vi "Z-Scan.vi"() -> ()   [LabVIEW 2010]
uses:
  <vilib>/Utility/error.llb/DialogType.ctl
  <vilib>/express/express arith-compare/Formula/XNode/ExpressFormulaBlockNode.xnode
  <vilib>/DAQmx/read.llb/DAQmx Read (Analog 1D Wfm NChan NSamp).vi
  <vilib>/DAQmx/create/channels.llb/DAQmx Create Channel (AI-Voltage-Basic).vi
  <vilib>/DAQmx/configure/timing.llb/DAQmx Timing (Sample Clock).vi
  <vilib>/DAQmx/configure/trigger.llb/DAQmx Start Trigger (Digital Edge).vi
  <vilib>/daqmx/miscellaneous.llb/DAQmx Fill In Error Info.vi
  <vilib>/express/express shared/transition.llb/Dynamic To Waveform Array.vi
  <vilib>/express/express shared/transition.llb/Waveform Array To Dynamic.vi
  <vilib>/express/express arith-compare/Formula/Block/exnFormulaBlock how many pts in the wave.vi
  <vilib>/express/express shared/ex_Modify Signal Name.vi
  Program Files (x86)/National Instruments/LabVIEW 2010/resource/objmgr/daqmx.rc
panel:
  in  "lower threshold":dbl
  in  "upper threshold":dbl
  out "Ioa":cluster{dbl[], dbl[]}(graph)
  in  "stop 11":bool
  out "Ica":cluster{dbl[], dbl[]}(graph)
  out "Ioca":cluster{dbl[], dbl[]}(graph)
  in  "x max (mm)":dbl=500.0
  in  "x step (mm)":dbl=5.0
  in  "N":i32=1000
  in  "x min (mm)":dbl=-0.5
  in  "error in":errorcluster
  out "Signal 2":waveform(dbl)[](graph)
  in  "Ring":u16(ring)=1 items=["Ref", "OA", "CA"]
  in  "stop 2":bool
  out "Trigger delay":dbl format="%#_6e"
  in  "Signal":tag="Dev2/ai0"
  in  "Minimum value (V)":dbl=-5.0
  in  "Maximum value (V)":dbl=10.0
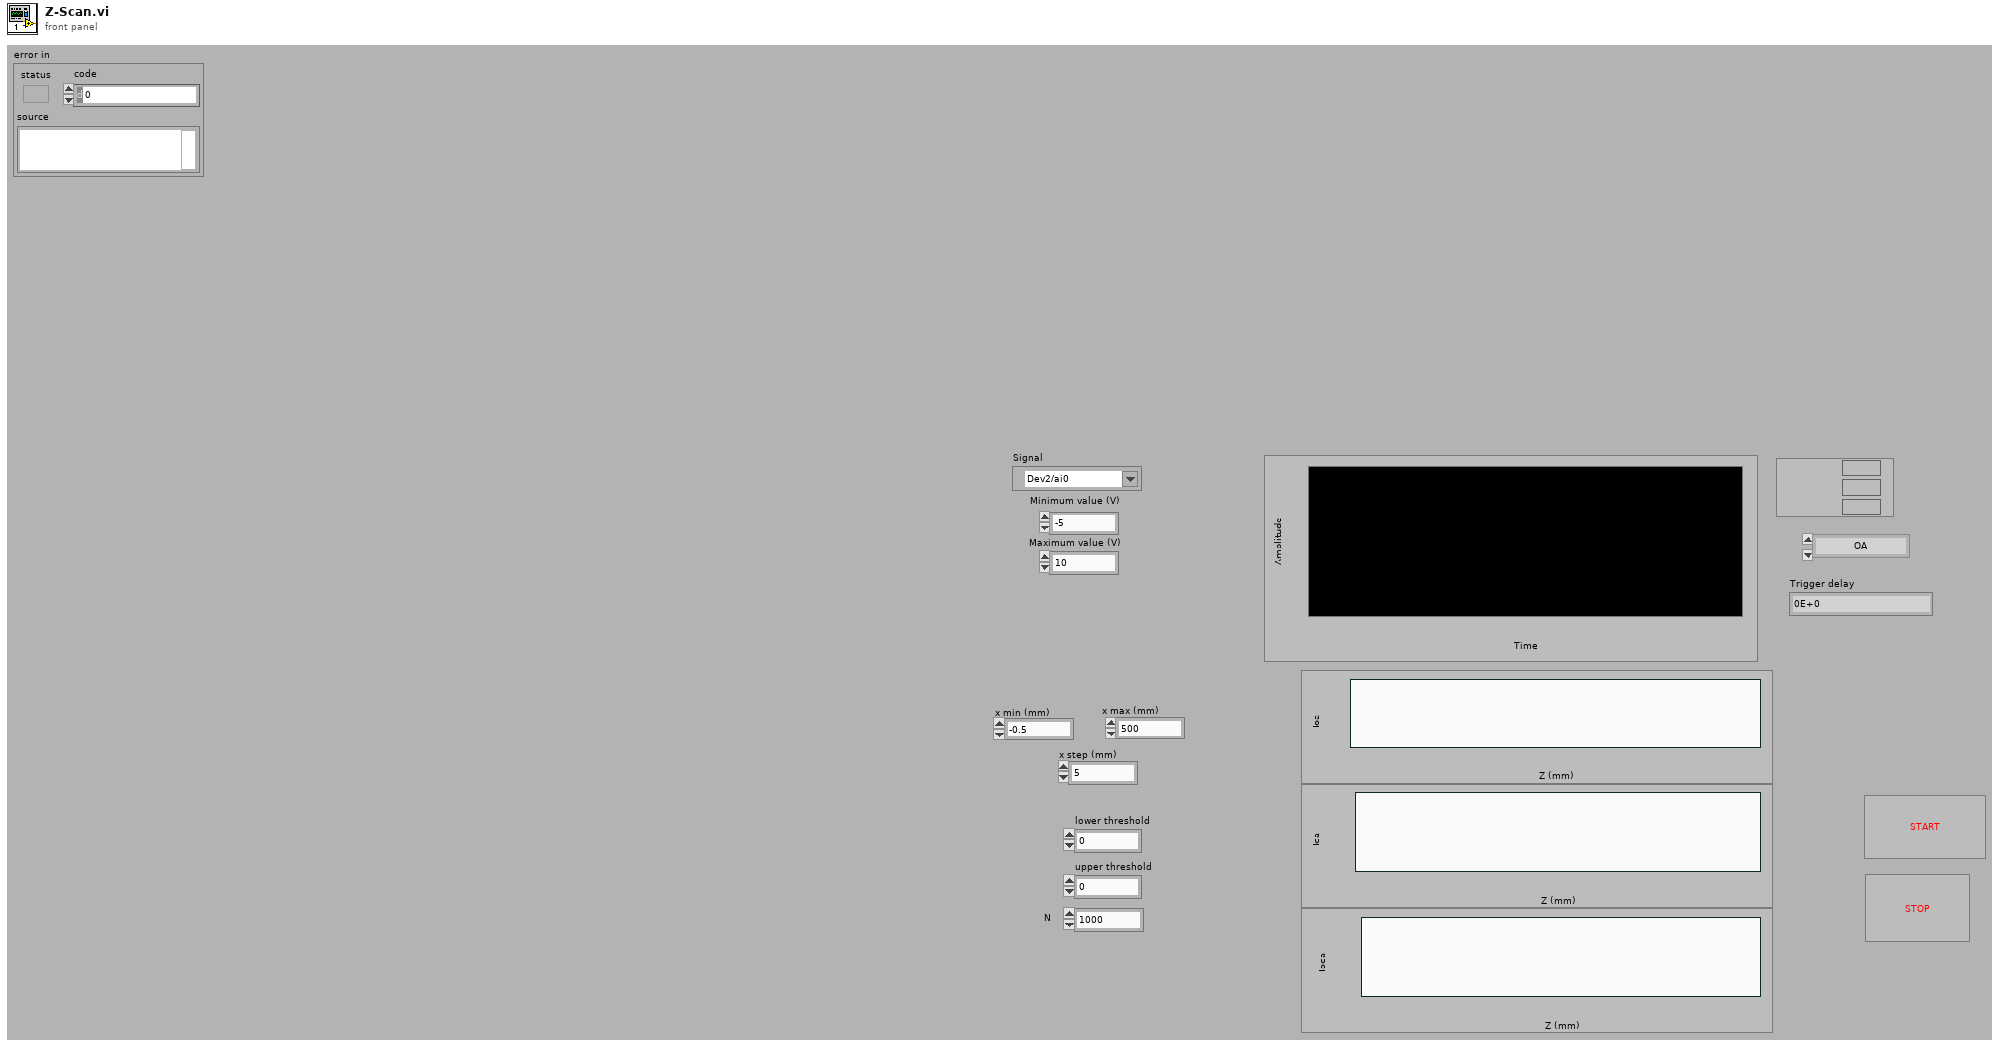
[diagram p1: front panel]
types:
  T1 = enum16{"open", "replace", "create", "open or create", "replace or create", "replace or create with confirmation"}
  T2 = typedef "DialogType.ctl" = u16
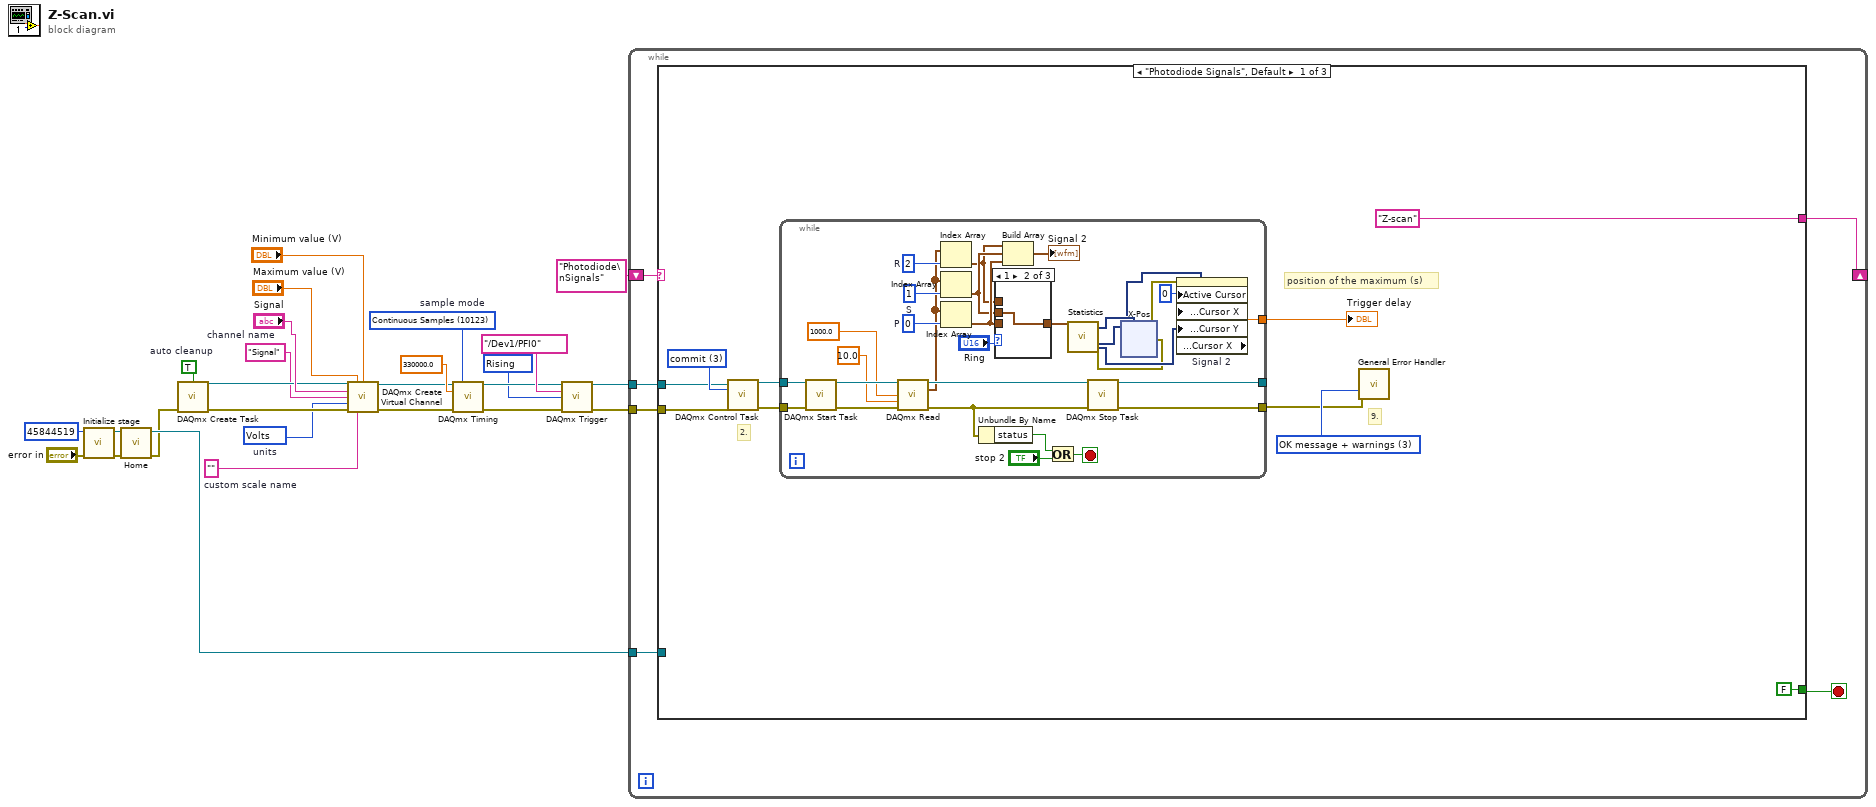
[diagram p0: block diagram]
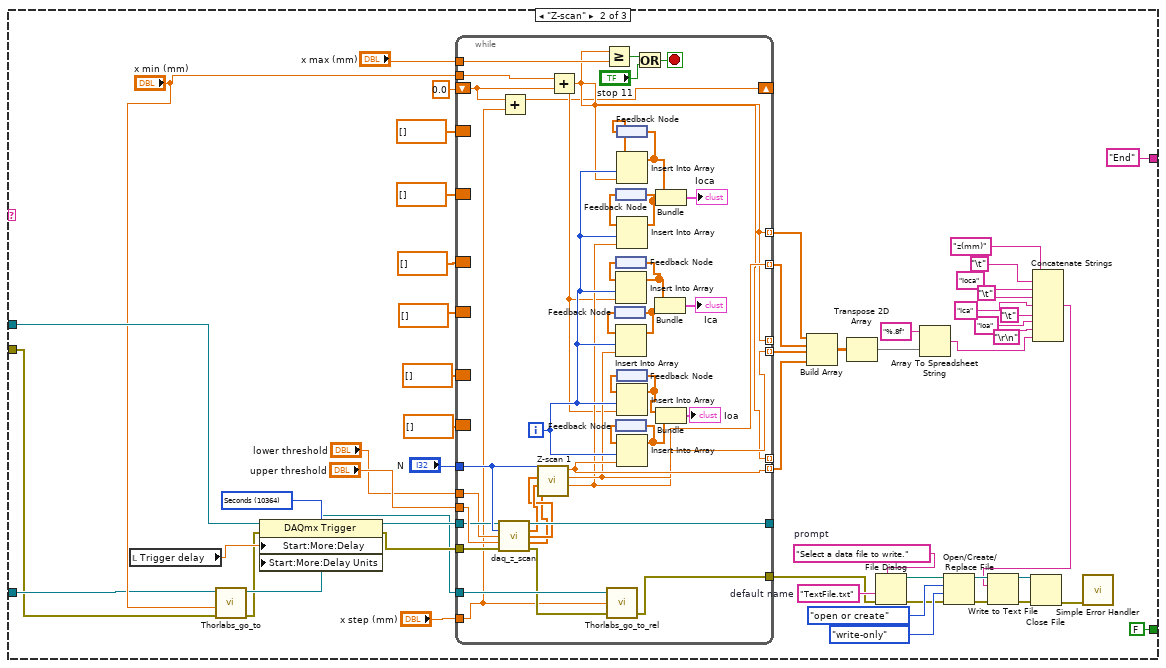
[diagram p4: hidden frame]
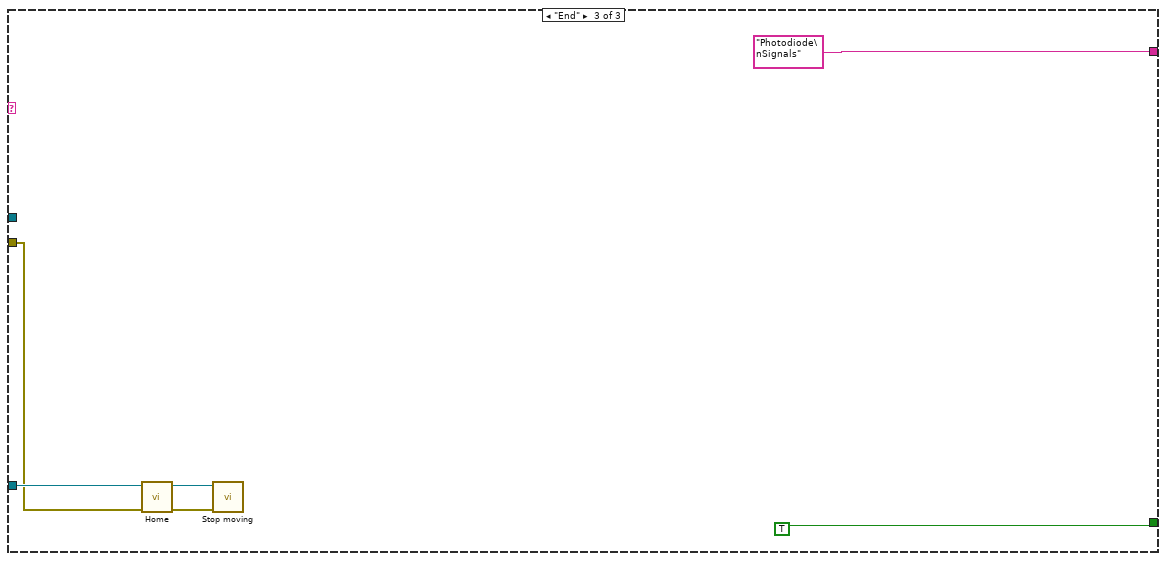
[diagram p5: hidden frame]
diagram:
  w15 = 10280 items=["Rising"=10280, "Falling"=10171] ("Trigger edge")
  w17 = 10123 items=["Finite Samples"=10178, "Continuous Samples"=10123, "Hardware Timed Single Point"=12522]  # sample mode
  w9 = 10348 items=["Volts"=10348, "From Custom Scale"=10065]  # units
  w10 = "Signal"  # channel name
  w8 = ""  # custom scale name
  w11 = TRUE  # auto cleanup
  n1 = call <instrlib>:"Initialize stage.vi"("error in (no error)"="error in", "HWSerialNum"=45844519) -> ("error out"=w6:errorcluster, "reference out"=w5:refnum<k7>)  [unwired: 8 in]
  n2 = call <instrlib>:"Home.vi"("error in"=w6, "in"=w5) -> ("error out"=w1:errorcluster, "out"=w2:refnum<k7>)  [unwired: 8 in]
  n3 = call <vilib>:"DAQmx Create Task.vi"("auto cleanup"=w11, "error in"=w1) -> ("task out"=w12:refnum<k21>, "error out"=w14:errorcluster)  [unwired: 12 in]
  n4 = call-poly <vilib>:"DAQmx Create Virtual Channel.vi"("task in"=w12, "maximum value"="Maximum value (V)", "minimum value"="Minimum value (V)", "physical channels"="Signal", "name to assign"=w10, "units"=w9, "error in"=w14, "custom scale name"=w8) -> ("task out"=w22:refnum<k21>, "error out"=w23:errorcluster)  [unwired: 6 in]
  n5 = call-poly <vilib>:"DAQmx Timing.vi"("task/channels in"=w22, "sample mode"=w17, "rate"=330000.0, "error in"=w23) -> ("task out"=w16:refnum<k21>, "error out"=w19:errorcluster)  [unwired: 10 in]
  n6 = call-poly <vilib>:"DAQmx Trigger.vi"("task/channels in"=w16, "source"=tag "/Dev1/PFI0", "edge"=w15, "error in"=w19) -> ("task out"=w26:refnum<k21>, "error out"=w25:errorcluster)  [unwired: 10 in]
  n7 = while {
    shift-right: [w31] -> _
    shift-left: "Photodiode\nSignals" -> [w32]
    tunnel: w26 -> [w30]
    tunnel: w25 -> [w29]
    tunnel: w2 -> [w27]
    stop <- w28 stop-if-true
    n8 = case shown="\"Photodiode Signals\", Default" w32 {
      tunnel: ["Z-scan" "End" "Photodiode\nSignals"] -> w31
      tunnel: w30 -> [w35 w252 _]
      tunnel: w29 -> [w34 w227 w310]
      tunnel: [FALSE FALSE TRUE] -> w28
      tunnel: w27 -> [_ w229 w312]
      frame "Photodiode Signals", Default {
        w41 = T2 3 items=["no dialog", "OK message", "continue or stop message", "OK message + warnings", "continue/stop + warnings"] ("type of dialog (OK msg:1)")
        w36 = 3 items=["verify"=2, "reserve"=4, "commit"=3, "unreserve"=5, "abort"=6] ("action")
        # "position of the maximum (s)"
        # "9."
        # "2."
        n9 = call <vilib>:"DAQmx Control Task.vi"("task/channels in"=w35, "action"=w36, "error in"=w34) -> ("task out"=w37:refnum<k21>, "error out"=w38:errorcluster)  [unwired: 11 in]
        n10 = while {
          tunnel: w37 -> [w73]
          tunnel: w38 -> [w72]
          tunnel: [w71] -> w40
          tunnel: [w49] -> _
          tunnel: [w48] -> w39
          stop <- w44 stop-if-true
          w64 = 0  # P
          w65 = 1  # S
          w66 = 2  # R
          n11 = call <vilib>:"DAQmx Start Task.vi"("task/channels in"=w73, "error in"=w72) -> ("task out"=w70:refnum<k21>, "error out"=w69:errorcluster)  [unwired: 12 in]
          n12 = call-poly <vilib>:"DAQmx Read.vi"("task/channels in"=w70, "number of samples per channel"=1000.0 ("Samples/channel"), "timeout"=10.0, "error in"=w69) -> ("task out"=w68:refnum<k21>, "data"=w63:waveform(dbl)[], "error out"=w46:errorcluster)  [unwired: 9 in]
          n13 = Index Array(array=w63, index=w66) -> (element=w55:waveform(dbl))
          n14 = Index Array(array=w63, index=w65) -> (element=w56:waveform(dbl))
          n15 = Index Array(array=w63, index=w64) -> (element=w58:waveform(dbl))
          n16 = Unbundle By Name(w46) -> ("status"=w47:bool)
          n17 = case shown="1" "Ring" {
            tunnel: w58 -> [w213 _ _]
            tunnel: [w213 w214 w215] -> w57
            tunnel: w56 -> [_ w214 _]
            tunnel: w55 -> [_ _ w215]
            frame 0, Default {
            }
            frame 1 {
            }
            frame 2 {
            }
          }
          n18 = Build Array(w55, w56, w58) -> (→"Signal 2":waveform(dbl)[])
          n19 = Or(x=w47, y="stop 2") -> (x .or. y?=w44:bool)
          n20 = call "Statistics"("Signals"=w57) -> ("First Time"=w60:dynamicdata, "Time of Maximum"=w61:dynamicdata, "Maximum"=w59:dynamicdata, "error out"=w54:errorcluster)  [unwired: 21 in, 2 out]
          n21 = call <vilib>:"DAQmx Stop Task.vi"("task/channels in"=w68, "error in"=w46) -> ("task out"=w49:refnum<k21>, "error out"=w48:errorcluster)  [unwired: 12 in]
          n22 = xnode "X-Pos"("TimeMax"=w61, "1stTime"=w60, "error in (no error)"=w54) -> ("Result"=w50:dynamicdata, "error out"=w53:errorcluster)
          n23 = property on="Signal 2" class="WFGraph (strict)"(error in=w53, "Active Cursor"=u32 0, "Cursor.Cursor Position:Cursor X"=w50, "Cursor.Cursor Position:Cursor Y"=w59) -> ("Cursor.Cursor Position:Cursor X"=w71:dbl)  [unwired: 1 in, 2 out]
        }
        "Trigger delay" <- w40
        n24 = call <vilib>:"General Error Handler.vi"("type of dialog (OK msg:1)"=w41, "error in (no error)"=w39) -> ()  [unwired: 9 in, 5 out]
      }
      frame "Z-scan" {
        w243 = "TextFile.txt"  # default name
        w244 = "Select a data file to write."  # prompt
        w255 = 10364 items=["Sample Clock Periods"=10286, "Seconds"=10364, "Ticks"=10304] ("Start.DelayUnits")
        n25 = local read "Trigger delay"() -> (w251:dbl)
        n26 = call <userlib>:"Thorlabs_go_to.vi"("error in (no error)"=w227, "Target position (mm)"="x min (mm)", "MG17Motor in"=w229) -> ("error out"=w226:errorcluster, "MG17Motor out"=w228:refnum<k7>)  [unwired: 6 in, 1 out]
        n27 = property class="DAQmx Trigger"(reference=w252, error in=w226, "Start:More:Delay"=w251, "Start:More:Delay Units"=w255) -> (reference out=w254:refnum<k21>, error out=w253:errorcluster)
        n28 = while {
          tunnel: "x max (mm)" -> [w303]
          tunnel: [w275] -> _ mode=indexing
          tunnel: [w296] -> w234 mode=indexing
          tunnel: [w271] -> w238
          tunnel: [w298] -> _
          tunnel: "x min (mm)" -> [w299]
          tunnel: "x step (mm)" -> [w269]
          tunnel: w228 -> [w295]
          tunnel: "N" -> [w297]
          shift-right: [w270] -> _
          shift-left: 0.0 -> [w292]
          border: dbl[] [] -> [_]
          border: dbl[] [] -> [_]
          tunnel: w253 -> [w273]
          tunnel: "upper threshold" -> [w294]
          tunnel: w254 -> [w293]
          border: dbl[] [] -> [_]
          border: dbl[] [] -> [_]
          border: dbl[] [] -> [_]
          border: dbl[] [] -> [_]
          tunnel: [w277] -> w235 mode=indexing
          tunnel: [w275] -> _ mode=indexing
          tunnel: [w276] -> w236 mode=indexing
          tunnel: [w275] -> w237 mode=indexing
          tunnel: "lower threshold" -> [w274]
          i -> [w281]
          stop <- w301 stop-if-true
          n29 = call <userlib>:"daq_z_scan.vi"("channels in"=w293, "N"=w297, "lower threshold"=w274, "upper threshold"=w294, "error in"=w273) -> ("task out"=w298:refnum<k21>, "CA"=w291:dbl[], "OA"=w290:dbl[], "Ref"=w289:dbl[], "error out"=w272:errorcluster)  [unwired: 6 in]
          n30 = Add(x=w292, y=w269) -> (x+y=w270:dbl)
          n31 = call <userlib>:"Z-scan 1.vi"("Ref"=w289, "CA"=w291, "OA"=w290, "N"=w297) -> ("Ioca"=w276:dbl, "Ica"=w277:dbl, "Ioa"=w296:dbl)  [unwired: 3 in]
          n32 = Add(x=w299, y=w292) -> (x+y=w275:dbl)
          n33 = Greater Or Equal?(x=w275, y=w303) -> (x >= y?=w302:bool)
          n34 = call <userlib>:"Thorlabs_go_to_rel.vi"("error in (no error)"=w272, "Step (mm)"=w269, "MG17Motor in"=w295) -> ("error out"=w271:errorcluster)  [unwired: 2 out]
          n35 = feedback #1() -> (w288:dbl[])
          n36 = feedback #2() -> (w279:dbl[])
          n37 = feedback #3() -> (w285:dbl[])
          n38 = Insert Into Array(array=w285, index=w281, new element=w275) -> (w286:dbl[])
          n39 = feedback-in #3(w286) -> ()
          n40 = Insert Into Array(array=w288, index=w281, new element=w277) -> (w287:dbl[])
          n41 = feedback-in #1(w287) -> ()
          n42 = feedback #4() -> (w306:dbl[])
          n43 = feedback #5() -> (w280:dbl[])
          n44 = Insert Into Array(array=w280, index=w281, new element=w275) -> (w282:dbl[])
          n45 = feedback-in #5(w282) -> ()
          n46 = Insert Into Array(array=w279, index=w281, new element=w276) -> (w283:dbl[])
          n47 = feedback-in #2(w283) -> ()
          n48 = feedback #6() -> (w307:dbl[])
          n49 = Insert Into Array(array=w307, index=w281, new element=w275) -> (w304:dbl[])
          n50 = feedback-in #6(w304) -> ()
          n51 = Insert Into Array(array=w306, index=w281, new element=w296) -> (w305:dbl[])
          n52 = feedback-in #4(w305) -> ()
          n53 = Or(x=w302, y="stop 11") -> (x .or. y?=w301:bool)
          n54 = Bundle(w286, w287) -> (→"Ica":cluster{dbl[], dbl[]})  [unwired: 1 in]
          n55 = Bundle(w282, w283) -> (→"Ioca":cluster{dbl[], dbl[]})  [unwired: 1 in]
          n56 = Bundle(w304, w305) -> (→"Ioa":cluster{dbl[], dbl[]})  [unwired: 1 in]
        }
        n57 = Build Array(w237, w236, w235, w234) -> (w233:dbl[][])
        n58 = Transpose 2D Array(2D array=w233) -> (transposed array=w232:dbl[][])
        n59 = File Dialog(7:w244, 8:w238, 9:w243) -> (0:w245:errorcluster, 3:w242:path)  [unwired: 6 out]
        n60 = Array To Spreadsheet String(array=w232, 3:"%.8f") -> (spreadsheet string=w217:string)  [unwired: 1 out]
        n61 = Open/Create/Replace File(file path (use dialog)=w242, error in=w245, operation (0:open)=T1."open or create", access (0:read/write)=enum16{"read/write", "read-only", "write-only"}."write-only") -> (refnum out=w246:refnum<file>, error out=w247:errorcluster)  [unwired: 3 out]
        n62 = Concatenate Strings("z(mm)", "\t", "Ioca", "\t", "Ica", "\t", "Ioa", "\r\n", w217) -> (w216:string)
        n63 = Write to Text File(file (use dialog)=w246, text=w216, error in=w247) -> (refnum out=w239:refnum<file>, error out=w240:errorcluster)  [unwired: 1 in, 1 out]
        n64 = Close File(refnum=w239, error in=w240) -> (error out=w241:errorcluster)  [unwired: 1 out]
        n65 = call <vilib>:"Simple Error Handler.vi"("error in (no error)"=w241) -> ()  [unwired: 1 in, 8 out]
      }
      frame "End" {
        n66 = call <instrlib>:"Home.vi"("error in"=w310, "in"=w312) -> ("error out"=w309:errorcluster, "out"=w311:refnum<k7>)  [unwired: 8 in]
        n67 = call <instrlib>:"Stop moving.vi"("error in (no error)"=w309, "Motor in"=w311) -> ()  [unwired: 8 in, 2 out]
      }
    }
  }
